vi "Update CLFNs.vi"() -> ()   [LabVIEW 2026]
uses:
  <vilib>/Utility/traverseref.llb/TRef TravTarget.ctl
  <vilib>/Utility/traverseref.llb/VI Scripting - Traverse.lvlib
panel:
  out "Array 2":string[](array[string])
  out "Array":string[](array[string])
  in  "Path":path
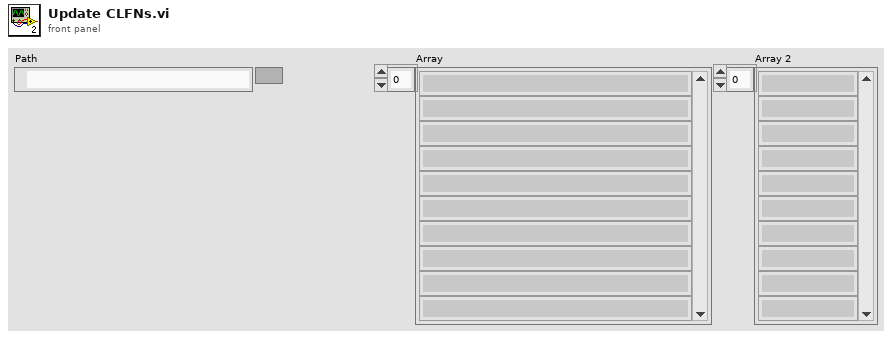
[diagram p1: front panel]
types:
  T1 = typedef "TRef TravTarget.ctl" = enum16{"FP", "BD", "Other"}
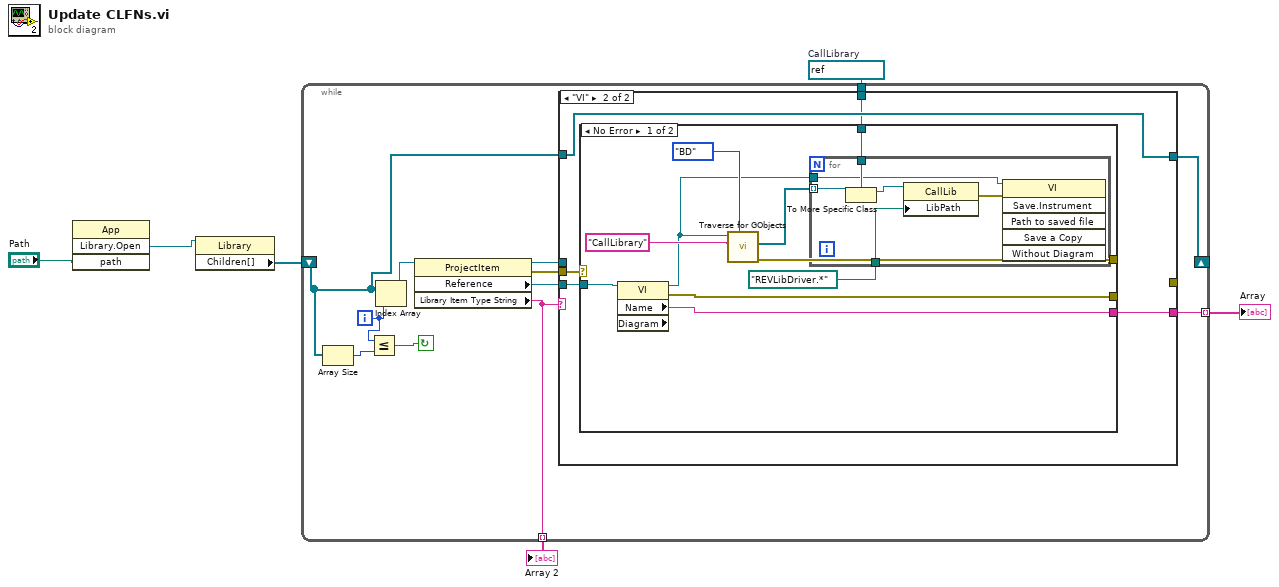
[diagram p0: block diagram]
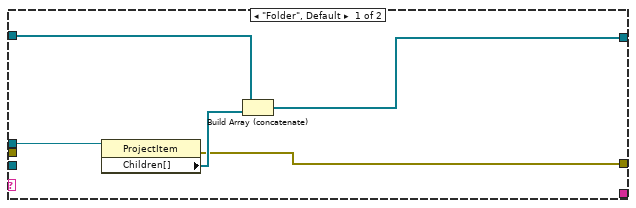
[diagram p2: hidden frame]
diagram:
  w1 = refnum<vi> refnum  # CallLibrary
  n1 = invoke class="App" method="Library.Open"("path"="Path") -> ("Open Library"=w5:refnum<vi>)  [unwired: 3 in, 3 out]
  n2 = property class="Library"(reference=w5) -> ("Children[]"=w4:refnum<vi>[])  [unwired: 1 in, 2 out]
  n3 = while {
    tunnel: [w16] -> w3 mode=indexing
    tunnel: [w15] -> w2 mode=indexing
    shift-right: [w12] -> _
    shift-left: w4 -> [w11]
    tunnel: w1 -> [w7]
    i -> [w10]
    stop <- w8 continue-if-true
    n4 = Array Size(array=w11) -> (size(s)=w9:i32)
    n5 = Less Or Equal?(x=w10, y=w9) -> (x <= y?=w8:bool)
    n6 = Index Array(array=w11, index=w10) -> (element=w13:refnum<vi>)
    n7 = property class="ProjectItem"(reference=w13) -> (reference out=w14:refnum<vi>, error out=w18:errorcluster, "Reference"=w17:refnum<vi>, "Library Item Type String"=w15:string)  [unwired: 1 in]
    n8 = case shown="\"VI\"" w15 {
      tunnel: w18 -> [_ w28]
      tunnel: w17 -> [_ w27]
      tunnel: [_ w26] -> w16
      tunnel: w14 -> [w23 _]
      tunnel: w11 -> [w22 w25]
      tunnel: [w20 w25] -> w12
      tunnel: [w19 _] -> _
      tunnel: w7 -> [_ w24]
      frame "Folder", Default {
        n9 = property class="ProjectItem"(reference=w23) -> (error out=w19:errorcluster, "Children[]"=w21:refnum<vi>[])  [unwired: 1 in, 1 out]
        n10 = Build Array (concatenate)(w22, w21) -> (w20:refnum<vi>[])
      }
      frame "VI" {
        n11 = case shown="No Error" w28 {
          tunnel: w27 -> [w38 _]
          tunnel: [w37 _] -> w26
          tunnel: [w36 _] -> _
          tunnel: [w33 _] -> _
          tunnel: w24 -> [w31 _]
          frame No Error {
            n12 = property class="VI" props=["Name", "Diagram"](reference=w38) -> (reference out=w29:refnum<vi>, error out=w36:errorcluster, "Name"=w37:string)  [unwired: 1 in, 1 out]
            n13 = call <vilib>:"Traverse for GObjects.vi"("Traverse Target"=TRef_TravTarget."BD", "Class Name"="CallLibrary", "VI Refnum"=w29) -> ("error out"=w33:errorcluster, "References"=w32:refnum<vi>[])  [unwired: 5 in, 2 out]
            n14 = for {
              tunnel: w32 -> [w44] mode=indexing
              tunnel: w31 -> [w43]
              tunnel: path "REVLibDriver.*" ("Class Name") -> [w41]
              tunnel: w29 -> [w39]
              n15 = To More Specific Class(target class=w43, reference=w44) -> (specific class reference=w42:refnum<vi>)  [unwired: 1 in, 1 out]
              n16 = property class="CallLib"(reference=w42, "LibPath"=w41) -> (error out=w40:errorcluster)  [unwired: 1 in, 1 out]
              n17 = invoke class="VI" method="Save.Instrument"(reference=w39, error in=w40) -> ()  [unwired: 4 in, 6 out]
            }
          }
          frame Error {
          }
        }
      }
    }
  }
  "Array" <- w3
  "Array 2" <- w2
